vi "Create.vi"(8 "error in (no error)":errorcluster, 10 "Report Path":path) -> (0 "error out":errorcluster, 3 "Text Report":refnum<class "Text Report.lvclass">)   [LabVIEW 2020, in "Text Report.lvclass"]
uses:
  Text Report.lvclass
  Text Report.lvclass/Text Report.ctl
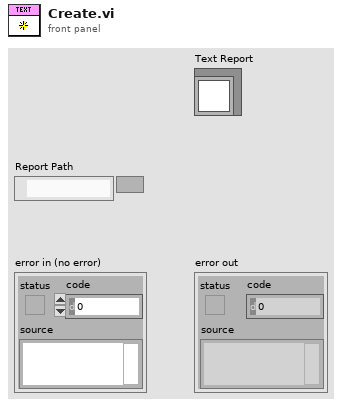
[diagram p1: front panel]
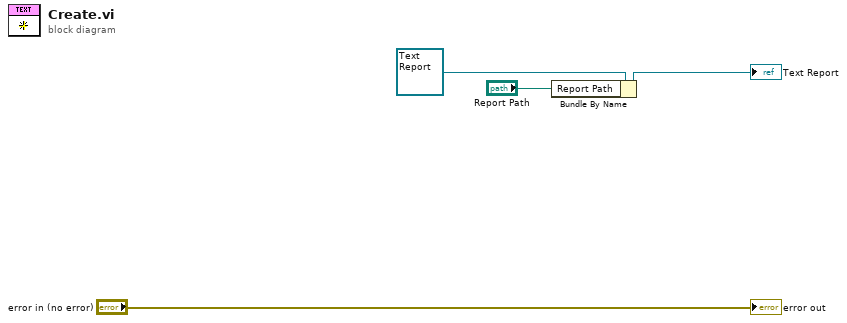
[diagram p0: block diagram]
diagram:
  n1 = Bundle By Name(cluster=refnum<class "Text Report.lvclass"> refnum ("Text Report"), "Report Path"="Report Path") -> (→"Text Report":refnum<class "Text Report.lvclass">)
  "error out" <- "error in (no error)"
